vi "toml_parse_name.vi"(8 "error in (no error)":errorcluster, 11 "string":string) -> (0 "error out":errorcluster, 2 "names":string[](array[string]), 3 "remaining string":string)   [LabVIEW 2017]
uses:
  <vilib>/Utility/error.llb/Error Cluster From Error Code.vi
  <vilib>/regexp/Match Regular Expression.xnode
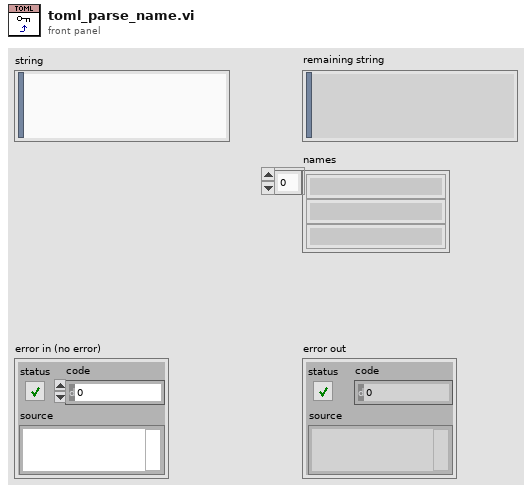
[diagram p1: front panel]
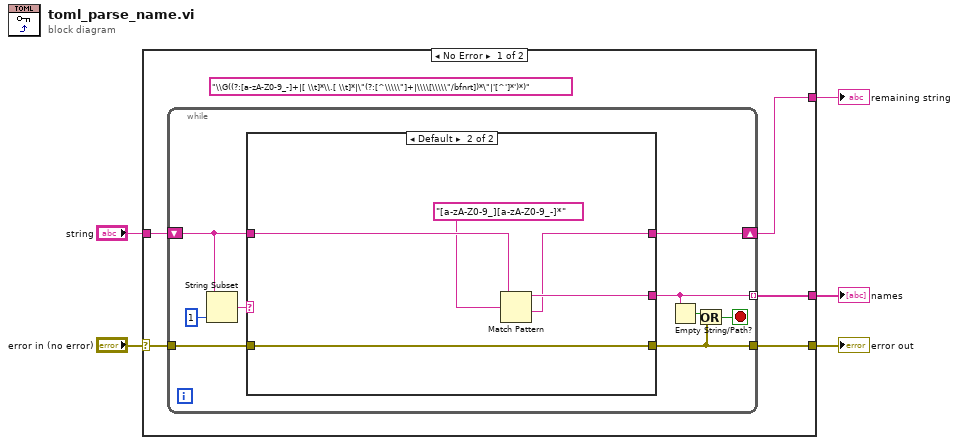
[diagram p0: block diagram]
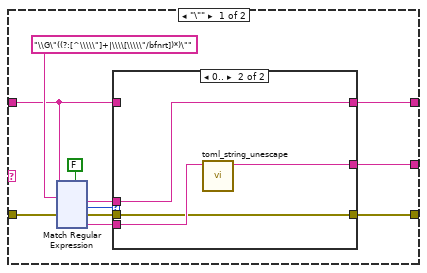
[diagram p2: hidden frame]
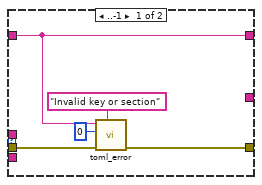
[diagram p3: hidden frame]
diagram:
  n1 = case shown="No Error" "error in (no error)" {
    selector: "error in (no error)" -> [w7 w162]
    tunnel: "string" -> [w9 w161]
    tunnel: [w6 w162] -> w3
    tunnel: [w8 w161] -> w2
    tunnel: [w10 _] -> w1
    frame No Error {
      (unwired) "\\G((?:[a-zA-Z0-9_-]+|[ \\t]*\\.[ \\t]*|\"(?:[^\\\\\"]+|\\\\[\\\\\"/bfnrt])*\"|'[^']*')*)"
      n2 = while {
        shift-right: [w16] -> w8
        shift-left: w9 -> [w18]
        tunnel: [w13] -> w10 mode=indexing
        tunnel: w7 -> [w14]
        tunnel: [w11] -> w6
        stop <- w12 stop-if-true
        n3 = String Subset(string=w18, length (rest)=1 ("length (rest)")) -> (substring=w17:string)  [unwired: 1 in]
        n4 = case shown="Default" w17 {
          tunnel: w18 -> [w22 w160]
          tunnel: [w26 w158] -> w13
          tunnel: [w24 w157] -> w16
          tunnel: w14 -> [w29 w156]
          tunnel: [w20 w156] -> w11
          frame "\"" {
            n5 = xnode "Match Regular Expression"("input string"=w22, "regular expression"="\\G\"((?:[^\\\\\"]+|\\\\[\\\\\"/bfnrt])*)\"", "error in"=w29, "multiline? (F)"=FALSE) -> ("after match"=w23:string, "offset past match"=w25:i32, "error out"=w21:errorcluster, "submatch 1"=w27:string)  [unwired: 2 in, 2 out]
            n6 = case shown="0.." w25 {
              tunnel: w27 -> [_ w39]
              tunnel: [_ w38] -> w26
              tunnel: [w33 w37] -> w24
              tunnel: w23 -> [_ w37]
              tunnel: w22 -> [w33 _]
              tunnel: w21 -> [w35 w36]
              tunnel: [w34 w36] -> w20
              frame ..-1 {
                n7 = call "toml_error.vi"("message"="Invalid key or section", "error in (no error)"=w35, "offset (0)"=0, "toml"=w33) -> ("error out"=w34:errorcluster)  [unwired: 7 in]
              }
              frame 0.. {
                n8 = call "toml_string_unescape.vi"("escaped string"=w39) -> ("string out"=w38:string)  [unwired: 9 in, 1 out]
              }
            }
          }
          frame Default {
            n9 = Match Pattern(string=w160, regular expression="[a-zA-Z0-9_][a-zA-Z0-9_-]*") -> (before substring=w158:string, after substring=w157:string)  [unwired: 1 in, 2 out]
          }
        }
        n10 = Empty String/Path?(string/path=w13) -> (empty?=w15:bool)
        n11 = Or(x=w15, y=w11) -> (x .or. y?=w12:bool)
      }
    }
    frame Error {
    }
  }
  "error out" <- w3
  "remaining string" <- w2
  "names" <- w1
